vi "Periodic Tasks.vi"() -> ()   [LabVIEW 2011]
doc: "This VI runs in parallel to other tasks. It can contain as many user-defined periodic loops as you need. These can carry out PID or other sorts of timed response."
uses:
  <vilib>/Rock Robotics/SystemInterfaces/Utilities/FPGA_UtilitiesLED State.ctl
  <vilib>/Rock Robotics/SystemInterfaces/Utilities/FPGA_UtilitiesLED Source.ctl
  <vilib>/Rock Robotics/WPI/Relay/WPI_RelayValue.ctl
  Robot Global Data.vi
panel:
  out "Direction":bool
  out "Distance":dbl
  in  "Home Speed":dbl=1.0
  in  "Home Position":dbl=2.85
  out "Current Voltage":dbl
  in  "upper limit":dbl=4.5
  in  "lower limit":dbl=0.85
  # "Speed to move to home"
  # "Target Tracking"
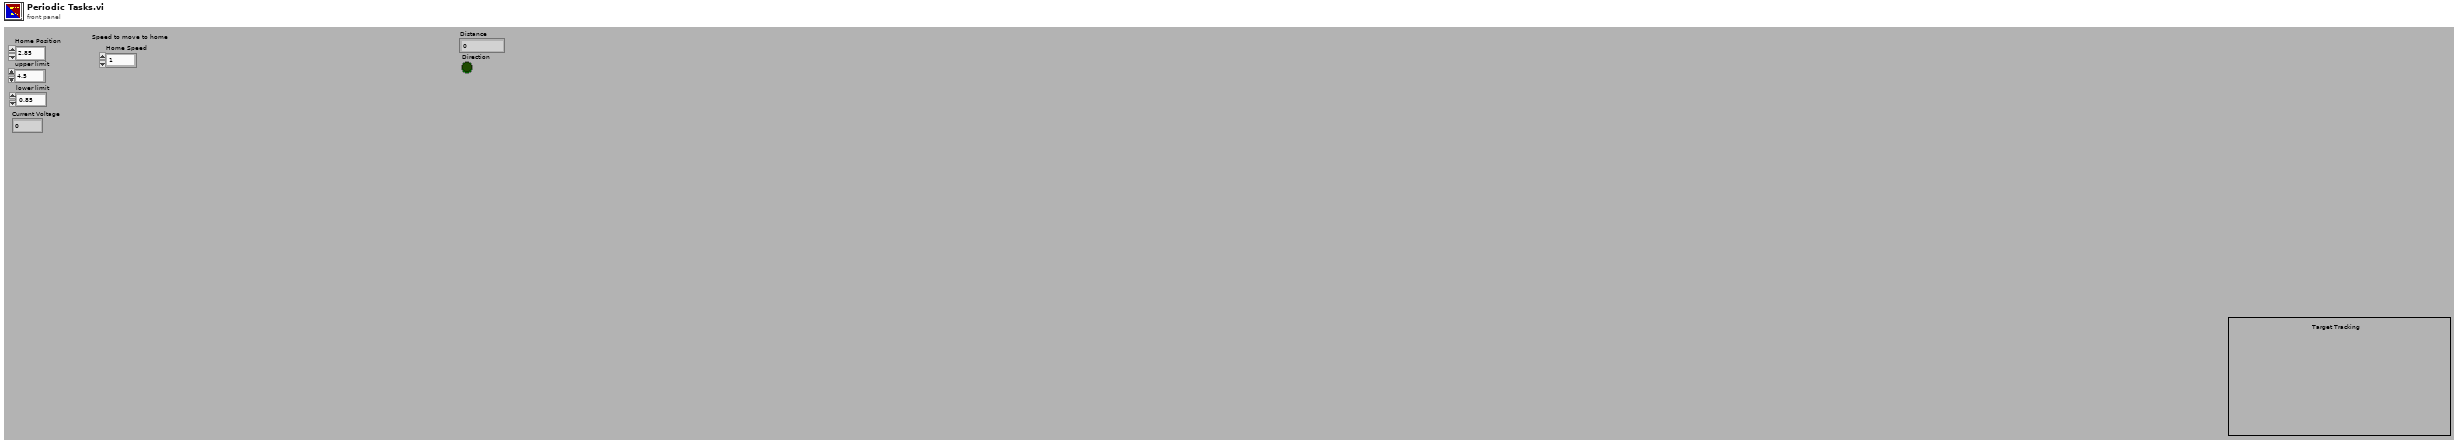
[diagram p1: front panel]
types:
  T1 = typedef "WPI_RelayValue.ctl" = enum16{"Off", "On", "Forward", "Reverse"}
  T2 = typedef "WPI_EncoderDevRef.ctl" = cluster{"DevStatus":errorcluster, "EncoderIndex":T3, "CounterIndex":T4, "DistancePerCount":dbl, "Decoding Type":T5}
  T3 = typedef "FPGA_EncoderIdx.ctl" = enum8{"Enc 0", "Enc 1", "Enc 2", "Enc 3", "Invalid"}
  T4 = typedef "FPGA_CounterCtrSystemIndex.ctl" = enum8{"Ctr 0", "Ctr 1", "Ctr 2", "Ctr 3", "Ctr 4", "Ctr 5", "Ctr 6", "Ctr 7", "Invalid"}
  T5 = typedef "WPI_EncoderType.ctl" = enum16{"1x", "2x", "4x"}
  T6 = typedef "WPI_AnalogChannelDevRef.ctl" = cluster{"DevStatus":errorcluster, "Analog Module":T7, "Analog Channel":T8}
  T7 = typedef "FPGA_TypedefAnalogModule.ctl" = enum16{"Analog Module 1", "Analog Module 2"}
  T8 = typedef "FPGA_AIChannel.ctl" = enum8{"AI 1", "AI 2", "AI 3", "AI 4", "AI 5", "AI 6", "AI 7", "AI 8", "Invalid"}
  T9 = typedef "WPI_RelayDevRef.ctl" = cluster{"DevStatus":errorcluster, "Relay Channel":T10, "Digital Module":T11, "Relay Direction":T12}
  T10 = typedef "FPGA_DIORelayChannel.ctl" = enum8{"Relay 1", "Relay 2", "Relay 3", "Relay 4", "Relay 5", "Relay 6", "Relay 7", "Relay 8", "Invalid"}
  T11 = typedef "FPGA_TypedefDigitalModule.ctl" = enum16{"Digital Module 1", "Digital Module 2"}
  T12 = typedef "WPI_RelayDirection.ctl" = enum16{"Both directions", "Forward only", "Reverse only"}
  T13 = cluster{"Driver Station Digital Output (1-8)[0]":bool, "Driver Station Digital Output (1-8)[1]":bool, "Driver Station Digital Output (1-8)[2]":bool, "Driver Station Digital Output (1-8)[3]":bool, "Driver Station Digital Output (1-8)[4]":bool, "Driver Station Digital Output (1-8)[5]":bool, "Driver Station Digital Output (1-8)[6]":bool, "Driver Station Digital Output (1-8)[7]":bool, "Driver Station Digital Output (1-8)[8]":bool}
  T14 = typedef "FPGA_UtilitiesLED State.ctl" = enum16{"Off", "On", "Toggle"}
  T15 = typedef "FPGA_UtilitiesLED Source.ctl" = enum16{"User LED", "FPGA LED"}
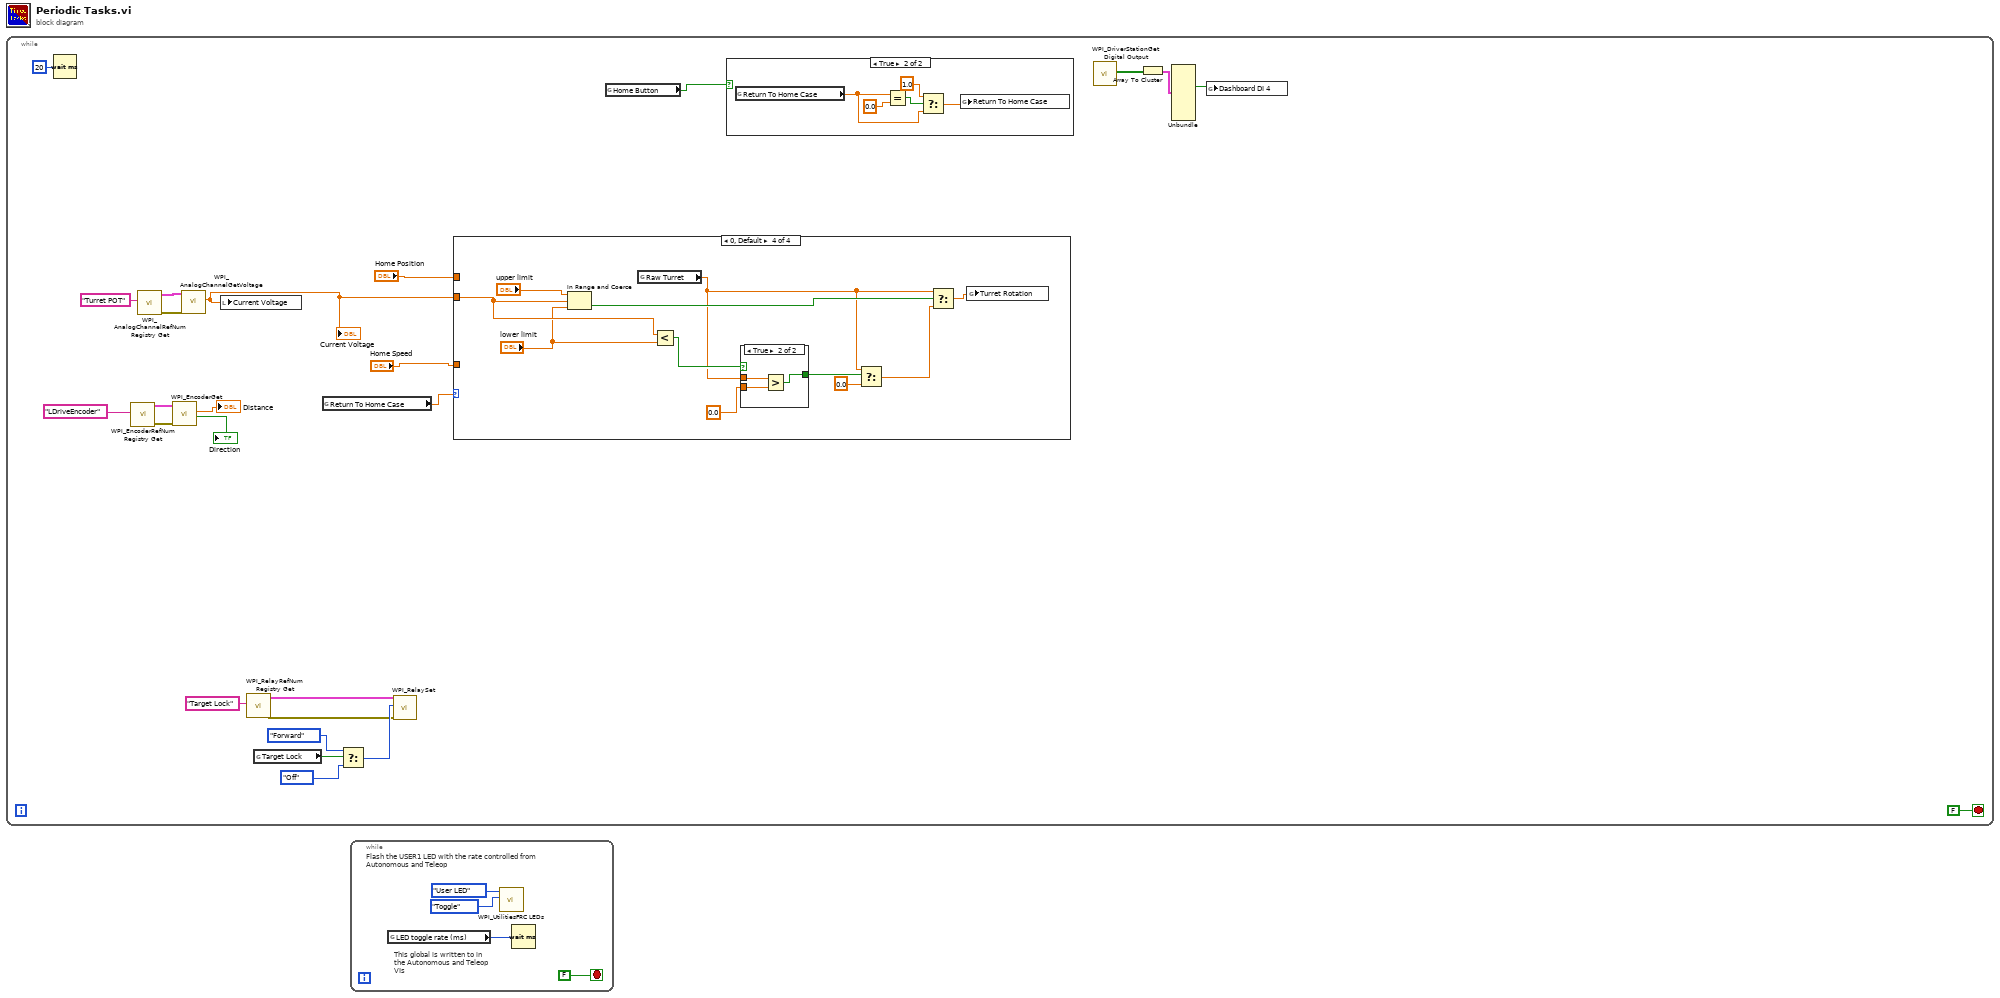
[diagram p0: block diagram]
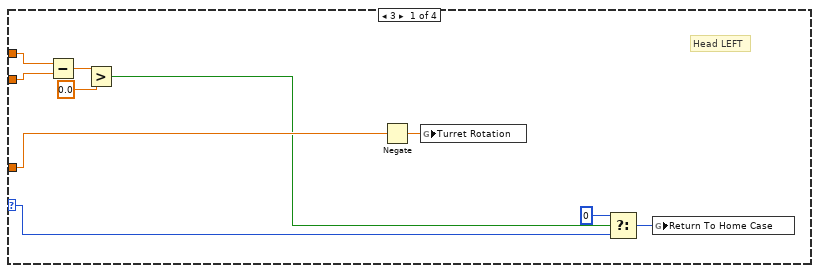
[diagram p2: hidden frame]
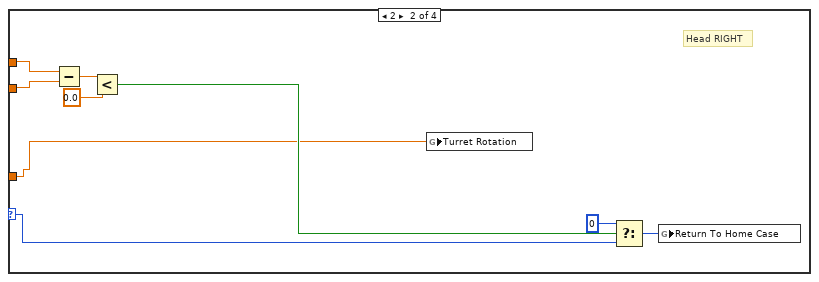
[diagram p3: hidden frame]
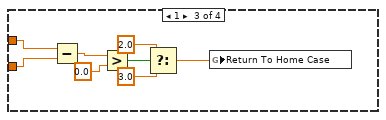
[diagram p4: hidden frame]
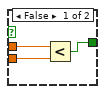
[diagram p5: hidden frame]
diagram:
  n1 = while {
    stop <- FALSE stop-if-true
    n2 = Wait (ms)(milliseconds to wait=u32 20) -> ()  [unwired: 1 out]
    n3 = call <vilib>:"WPI_EncoderRefNum Registry Get.vi"("refnum name"="LDriveEncoder") -> ("error out"=w2:errorcluster, "EncoderDevRef"=w3:T2)  [unwired: 9 in]
    n4 = call <vilib>:"WPI_AnalogChannelRefNum Registry Get.vi"("refnum name"="Turret POT") -> ("error out"=w5:errorcluster, "AIDeviceRef"=w6:T6)  [unwired: 9 in]
    n5 = call <vilib>:"WPI_EncoderGet.vi"("error in (no error)"=w2, "EncoderDevRef"=w3) -> ("Direction"=→"Direction":bool, "Distance"=→"Distance":dbl)  [unwired: 4 in, 4 out]
    n6 = call <vilib>:"WPI_AnalogChannelGetVoltage.vi"("error in (no error)"=w5, "AIDeviceRef"=w6) -> ("Voltage"=w14:dbl)  [unwired: 7 in, 2 out]
    "Current Voltage" <- w14
    n7 = local write "Current Voltage"(w14) -> ()
    n8 = call <vilib>:"WPI_RelayRefNum Registry Get.vi"("refnum name"="Target Lock") -> ("error out"=w16:errorcluster, "RelayDevRef"=w17:T9)  [unwired: 9 in]
    n9 = global read "Robot Global Data.vi" "Target Lock"() -> (w22:bool)
    n10 = global read "Robot Global Data.vi" "Return To Home Case"() -> (w13:dbl)
    n11 = Select(t=WPI_RelayValue."Forward" ("RelayValue"), s=w22, f=WPI_RelayValue."Off" ("RelayValue")) -> (s? t:f=w19:T1)
    n12 = call <vilib>:"WPI_RelaySet.vi"("error in (no error)"=w16, "RelayValue"=w19, "RelayDevRef"=w17) -> ()  [unwired: 7 in, 2 out]
    n13 = case shown="0, Default" w13 {
      selector: w13 -> [w33 w37 _ _]
      tunnel: w14 -> [w29 w38 w51 w63]
      tunnel: "Home Position" -> [w30 w39 w52 _]
      tunnel: "Home Speed" -> [w31 w36 _ _]
      frame 3 {
        # "Head LEFT"
        n14 = Subtract(x=w30, y=w29) -> (x-y=w28:dbl)
        n15 = Greater?(x=w28, y=0.0) -> (0:w26:bool)
        n16 = Negate(x=w31) -> (-x=w32:dbl)
        n17 = global write "Robot Global Data.vi" "Turret Rotation"(w32) -> ()
        n18 = Select(t=0, s=w26, f=w33) -> (s? t:f=w34:i32)
        n19 = global write "Robot Global Data.vi" "Return To Home Case"(w34) -> ()
      }
      frame 2 {
        # "Head RIGHT"
        n20 = Subtract(x=w39, y=w38) -> (x-y=w42:dbl)
        n21 = Less?(x=w42, y=0.0) -> (x < y?=w40:bool)
        n22 = global write "Robot Global Data.vi" "Turret Rotation"(w36) -> ()
        n23 = Select(t=0, s=w40, f=w37) -> (s? t:f=w43:i32)
        n24 = global write "Robot Global Data.vi" "Return To Home Case"(w43) -> ()
      }
      frame 1 {
        n25 = Subtract(x=w52, y=w51) -> (x-y=w50:dbl)
        n26 = Greater?(x=w50, y=0.0) -> (0:w48:bool)
        n27 = Select(t=2.0, s=w48, f=3.0) -> (s? t:f=w45:dbl)
        n28 = global write "Robot Global Data.vi" "Return To Home Case"(w45) -> ()
      }
      frame 0, Default {
        n29 = In Range and Coerce(upper limit="upper limit", x=w63, lower limit="lower limit") -> (In Range?=w60:bool)  [unwired: 1 out]
        n30 = global read "Robot Global Data.vi" "Raw Turret"() -> (w53:dbl)
        n31 = Less?(x=w63, y="lower limit") -> (x < y?=w55:bool)
        n32 = case shown="True" w55 {
          tunnel: 0.0 -> [w65 w69]
          tunnel: [w64 w68] -> w56
          tunnel: w53 -> [w66 w67]
          frame False {
            n33 = Less?(x=w66, y=w65) -> (x < y?=w64:bool)
          }
          frame True {
            n34 = Greater?(x=w67, y=w69) -> (0:w68:bool)
          }
        }
        n35 = Select(t=w53, s=w56, f=0.0) -> (s? t:f=w54:dbl)
        n36 = Select(t=w53, s=w60, f=w54) -> (s? t:f=w62:dbl)
        n37 = global write "Robot Global Data.vi" "Turret Rotation"(w62) -> ()
      }
    }
    n38 = global read "Robot Global Data.vi" "Home Button"() -> (w10:bool)
    n39 = case shown="True" w10 {
      frame False {
      }
      frame True {
        n40 = global read "Robot Global Data.vi" "Return To Home Case"() -> (w71:dbl)
        n41 = Equal?(x=w71, y=0.0) -> (x = y?=w73:bool)
        n42 = Select(t=1.0, s=w73, f=w71) -> (s? t:f=w70:dbl)
        n43 = global write "Robot Global Data.vi" "Return To Home Case"(w70) -> ()
      }
    }
    n44 = call <vilib>:"WPI_DriverStationGet Digital Output.vi"() -> ("Driver Station Digital Output (1-8)"=w25:bool[])  [unwired: 10 in, 1 out]
    n45 = Array To Cluster(array=w25) -> (cluster=w24:T13)
    n46 = Unbundle(w24) -> ("Driver Station Digital Output (1-8)[3]"=w23:bool)  [unwired: 8 out]
    n47 = global write "Robot Global Data.vi" "Dashboard DI 4"(w23) -> ()
  }
  n48 = while {
    stop <- FALSE stop-if-true
    # "This global is written to in the Autonomous and Teleop VIs"
    # "Flash the USER1 LED with the rate controlled from Autonomous and Teleop"
    n49 = global read "Robot Global Data.vi" "LED toggle rate (ms)"() -> (w75:u32)
    n50 = call <vilib>:"WPI_UtilitiesFRC LEDs.vi"("State"=FPGA_UtilitiesLED_State."Toggle", "LED Type"=FPGA_UtilitiesLED_Source."User LED") -> ()  [unwired: 1 in, 9 out]
    n51 = Wait (ms)(milliseconds to wait=w75) -> ()  [unwired: 1 out]
  }
